vi "Templates Directory.vi"(10 "Base Path":path) -> (2 "Templates Directory":path)   [LabVIEW 2021, in "_Template.lvlib"]
uses:
  _Template.lvlib
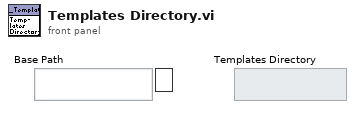
[diagram p1: front panel]
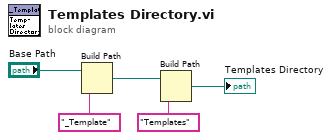
[diagram p0: block diagram]
diagram:
  n1 = Build Path(base path="Base Path", name or relative path="_Template" ("regular expression")) -> (appended path=w2:path)
  n2 = Build Path(base path=w2, name or relative path="Templates" ("regular expression")) -> (appended path=→"Templates Directory":path)
